vi "GFITS_NetServer.vi"(6 "port":u16, 7 "ID":string, 8 "error in (no error)":errorcluster, 9 "notifier In":refnum<notifier>, 10 "messages from sock":refnum<queue>, 11 "listener ID":refnum<k5>) -> (0 "error out":errorcluster)   [LabVIEW 2016]
uses:
  DHS_TCPSERVER_MsgStruct.ctl
panel:
  in  "ResponseStruct":T1
  out "sock ID":refnum<k5>
  out "stop":bool
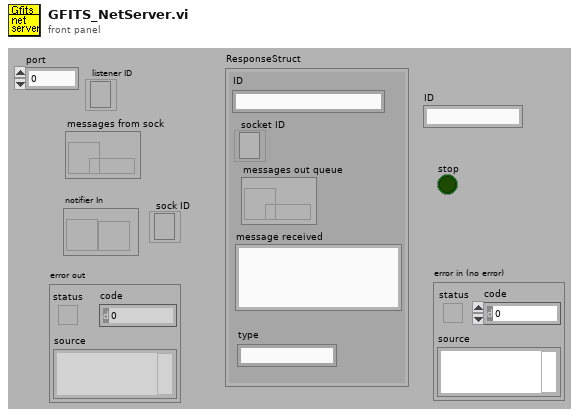
[diagram p1: front panel]
types:
  T1 = typedef "DHS_TCPSERVER_MsgStruct.ctl" = cluster{"ID":string, "socket ID":refnum<k5>, "messages out queue":refnum<queue>, "message received":string, "type":string}
  T2 = enum16{"Standard", "Buffered", "CRLF", "Immediate"}
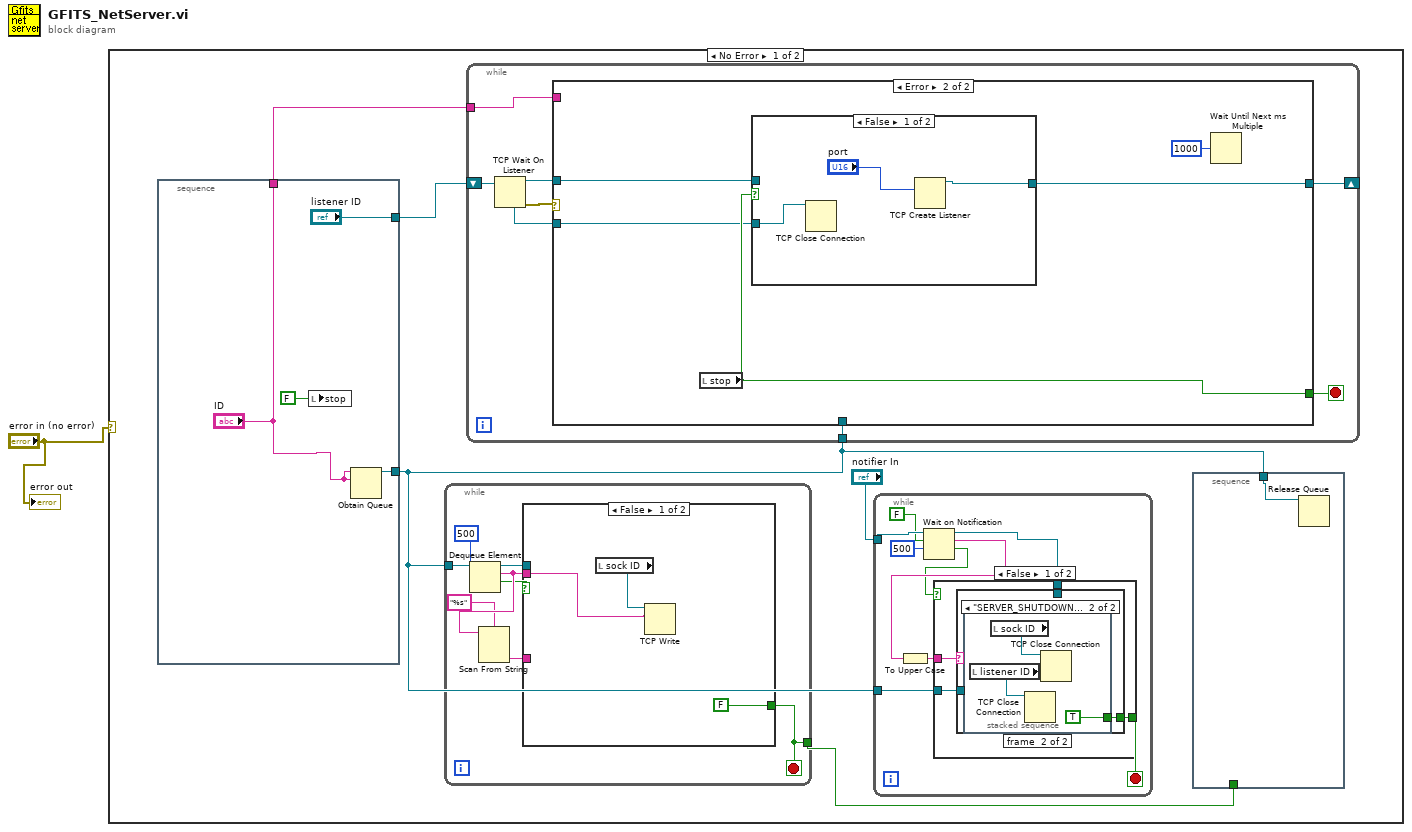
[diagram p0: block diagram]
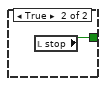
[diagram p2: hidden frame]
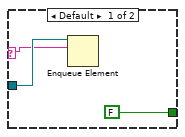
[diagram p3: hidden frame]
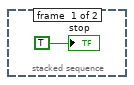
[diagram p4: hidden frame]
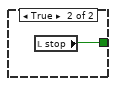
[diagram p5: hidden frame]
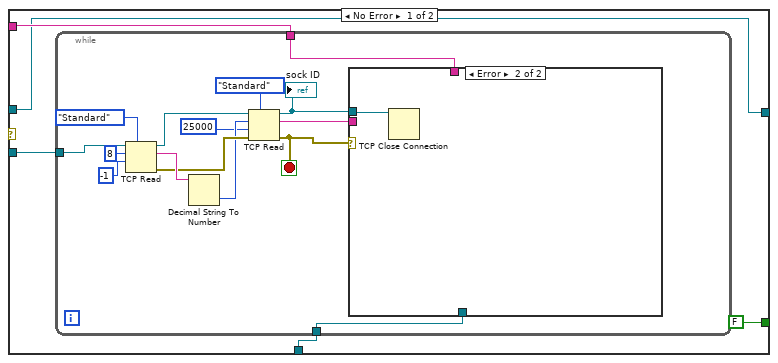
[diagram p6: hidden frame]
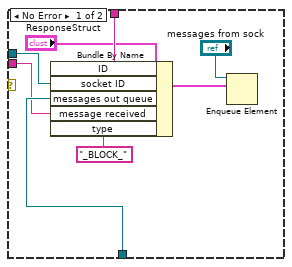
[diagram p7: hidden frame]
diagram:
  n1 = case shown="No Error" "error in (no error)" {
    frame No Error {
      n2 = stacked-sequence {
        tunnel: [w11] -> w3
        tunnel: ["listener ID"] -> w2
        tunnel: ["ID"] -> w5
        frame #0 {
          n3 = local write "stop"(FALSE ("stop")) -> ()
          n4 = Obtain Queue(name (unnamed)="ID", element data type="ID") -> (queue out=w11:refnum<queue>)  [unwired: 3 in, 2 out]
        }
      }
      n5 = while {
        tunnel: w3 -> [w19]
        tunnel: [w12] -> w4
        stop <- w12 stop-if-true
        n6 = Dequeue Element(queue=w19, timeout in ms (-1)=500) -> (queue out=w15:refnum<queue>, element=w18:string, timed out?=w14:bool)  [unwired: 1 in, 1 out]
        n7 = Scan From String(format string="%s", input string=w18) -> (output 1=w16:string)  [unwired: 2 in, 4 out]
        n8 = case shown="False" w14 {
          tunnel: w18 -> [w22 _]
          tunnel: w16 -> [_ _]
          tunnel: [FALSE w23] -> w12
          tunnel: w15 -> [_ _]
          frame False {
            n9 = local read "sock ID"() -> (w20:refnum<k5>)
            n10 = TCP Write(connection ID=w20, data in=w22) -> ()  [unwired: 1 in, 4 out]
          }
          frame True {
            n11 = local read "stop"() -> (w23:bool)
          }
        }
      }
      n12 = while {
        tunnel: w3 -> [w51]
        tunnel: w5 -> [w50]
        shift-right: [w47] -> _
        shift-left: w2 -> [w49]
        stop <- w46 stop-if-true
        n13 = TCP Wait On Listener(11:w49) -> (0:w53:errorcluster, 3:w48:refnum<k5>, 4:w52:refnum<k5>)  [unwired: 1 in, 4 out]
        n14 = case shown="Error" w53 {
          tunnel: w52 -> [w58 w83]
          tunnel: w51 -> [w57 _]
          tunnel: w50 -> [w56 _]
          tunnel: w48 -> [w55 w85]
          tunnel: [w55 w87] -> w47
          tunnel: [FALSE ("stop") w86] -> w46
          frame No Error {
            n15 = while {
              tunnel: w58 -> [w63]
              tunnel: w57 -> [w68]
              tunnel: w56 -> [w69]
              stop <- w72 stop-if-true
              n16 = TCP Read(connection ID=w63, bytes to read=8, 7:T2."Standard" ("mode (standard)"), 9:-1 ("timeout ms (25000)")) -> (connection ID out=w62:refnum<k5>, data out=w65:string, error out=w61:errorcluster)  [unwired: 1 in]
              n17 = Decimal String To Number(string=w65) -> (number=w60:i32)  [unwired: 3 out]
              n18 = TCP Read(connection ID=w62, bytes to read=w60, error in (no error)=w61, 7:T2."Standard" ("mode (standard)"), 9:25000 ("timeout ms (25000)")) -> (connection ID out=w70:refnum<k5>, data out=w71:string, error out=w72:errorcluster)
              "sock ID" <- w70
              n19 = case shown="Error" w72 {
                tunnel: w71 -> [w77 _]
                tunnel: w68 -> [w79 _]
                tunnel: w70 -> [w81 w82]
                tunnel: w69 -> [w80 _]
                frame No Error {
                  n20 = Bundle By Name(cluster="ResponseStruct", "ID"=w80, "socket ID"=w81, "messages out queue"=w79, "message received"=w77, "type"="_BLOCK_") -> (w74:T1)
                  n21 = Enqueue Element(queue="messages from sock", element=w74) -> ()  [unwired: 1 in, 4 out]
                }
                frame Error {
                  n22 = TCP Close Connection(connection ID=w82) -> ()  [unwired: 1 in, 3 out]
                }
              }
            }
          }
          frame Error {
            n23 = local read "stop"() -> (w86:bool)
            n24 = case shown="False" w86 {
              tunnel: [w89 w91] -> w87
              tunnel: w85 -> [_ w91]
              tunnel: w83 -> [w88 _]
              frame False {
                n25 = TCP Close Connection(connection ID=w88) -> ()  [unwired: 1 in, 3 out]
                n26 = TCP Create Listener(10:"port") -> (3:w89:refnum<k5>)  [unwired: 1 in, 5 out]
              }
              frame True {
              }
            }
            n27 = Wait Until Next ms Multiple(millisecond multiple=u32 1000) -> ()  [unwired: 1 out]
          }
        }
      }
      n28 = while {
        tunnel: "notifier In" -> [w32]
        tunnel: w3 -> [w27]
        stop <- w24 stop-if-true
        n29 = Wait on Notification(notifier=w32, ignore previous (F)=FALSE, timeout in ms (-1)=500) -> (notifier out=w30:refnum<notifier>, notification=w29:string, timed out?=w25:bool)  [unwired: 1 in, 1 out]
        n30 = To Upper Case(1:w29) -> (0:w28:string)
        n31 = case shown="False" w25 {
          tunnel: w30 -> [w36 _]
          tunnel: w28 -> [w35 _]
          tunnel: [w34 w45] -> w24
          tunnel: w27 -> [w33 _]
          frame False {
            n32 = case shown="\"SERVER_SHUTDOWN\"" w35 {
              selector: w35 -> [w37 _]
              tunnel: w36 -> [_ _]
              tunnel: [FALSE w40] -> w34
              tunnel: w33 -> [w38 _]
              frame Default {
                n33 = Enqueue Element(queue=w38, element=w37) -> ()  [unwired: 1 in, 4 out]
              }
              frame "SERVER_SHUTDOWN" {
                n34 = stacked-sequence {
                  tunnel: [_ TRUE] -> w40
                  frame #0 {
                    "stop" <- TRUE ("stop")
                  }
                  frame #1 {
                    n35 = local read "listener ID"() -> (w42:refnum<k5>)
                    n36 = local read "sock ID"() -> (w43:refnum<k5>)
                    n37 = TCP Close Connection(connection ID=w42) -> ()  [unwired: 1 in, 3 out]
                    n38 = TCP Close Connection(connection ID=w43) -> ()  [unwired: 1 in, 3 out]
                  }
                }
              }
            }
          }
          frame True {
            n39 = local read "stop"() -> (w45:bool)
          }
        }
      }
      n40 = stacked-sequence {
        tunnel: w4 -> [_]
        tunnel: w3 -> [w7]
        frame #0 {
          n41 = Release Queue(queue=w7) -> ()  [unwired: 1 in, 4 out]
        }
      }
    }
    frame Error {
    }
  }
  "error out" <- "error in (no error)"
